vi "Configure Acquisition.vi"(0 "VISA resource name":refnum<visa-resource-name>, 1 "Enable Analog Averaging (Disable)":bool, 2 "Number Of Averages (8)":i32=8, 5 "Acquisition Type (0: Normal)":i32(ring) items=["Normal", "Peak Detect", "High Resolution"], 7 "Sampling Mode  (0: Real Time)":i32(ring) items=["Real Time", "Equivalent Time", "Segment", "Real Time Peak Detect", "Real Time High Resolution", "Peak Detect Segment", "High Resolution Segment"], 9 "Interpolation (0:No Interpolation)":u32(ring) items=["No Interpolation", "sin(x)/x", "1 Point sin(x)/x", "2 Point sin(x)/x", "4 Point sin(x)/x", "8 Point sin(x)/x", "16 Point sin(x)/x"], 11 "error in (no error)":errorcluster, 12 "Segment Count (256)":i32=256, 13 "Resolution (0:Auto)":i32(ring) items=["Auto", "Bits 9", "Bits 10", "Bits 11", "Bits 12", "Fixed 11", "Fixed 12", "Fixed 13", "Fixed 14", "Fixed 15", "Fixed 16"]) -> (4 "VISA resource name out":refnum<visa-resource-name>, 15 "error out":errorcluster)   [LabVIEW 2020, in "Agilent 90000 Series.lvlib"]
doc: "Configures how the oscilloscope acquires data and fills the waveform record."
uses:
  Agilent 90000 Series.lvlib
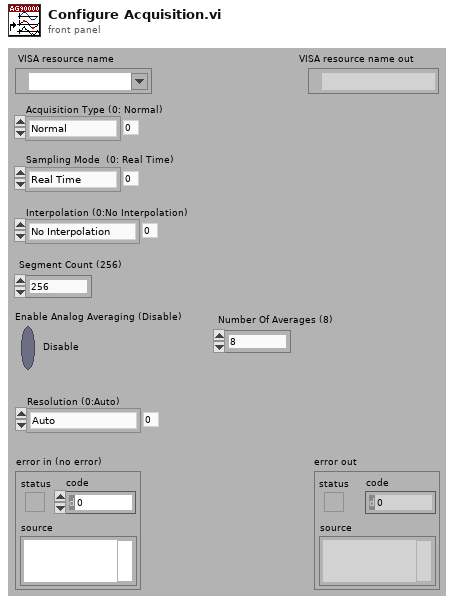
[diagram p1: front panel]
types:
  T1 = enum16{"Real Time", "Peak Detect", "High Resolution"}
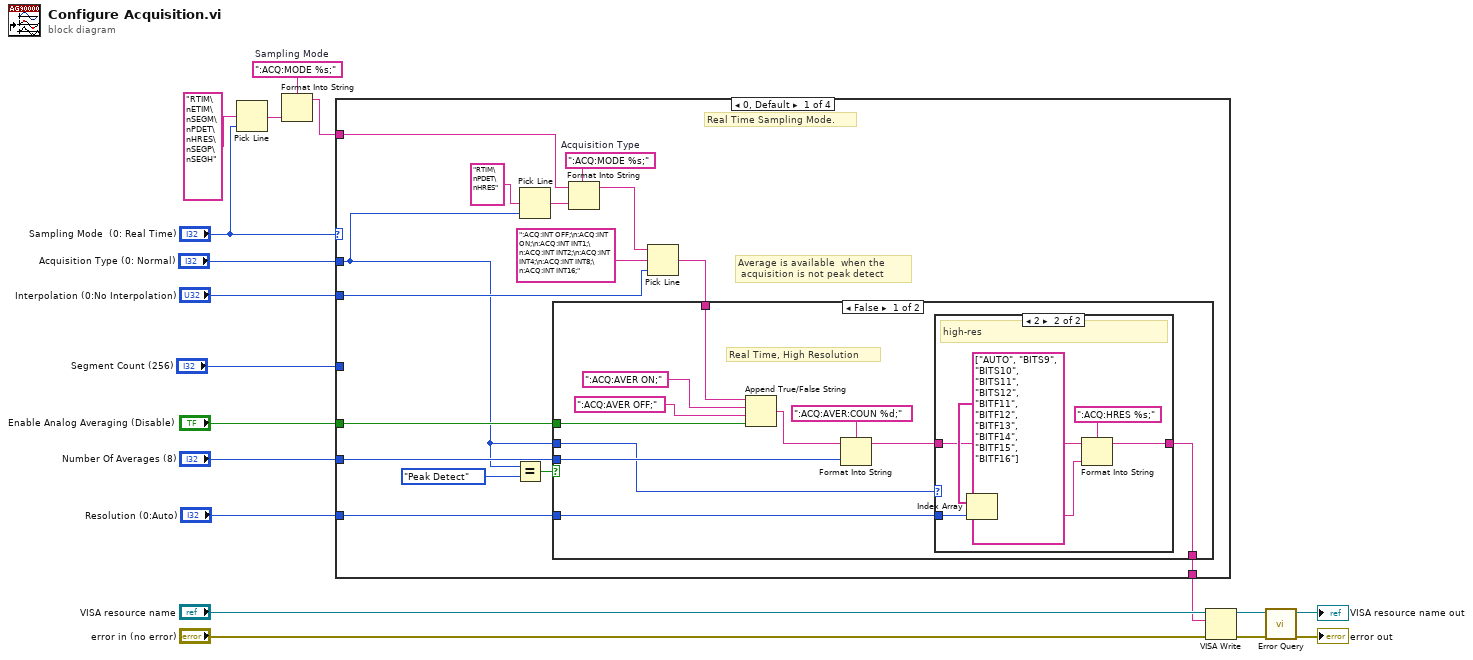
[diagram p0: block diagram]
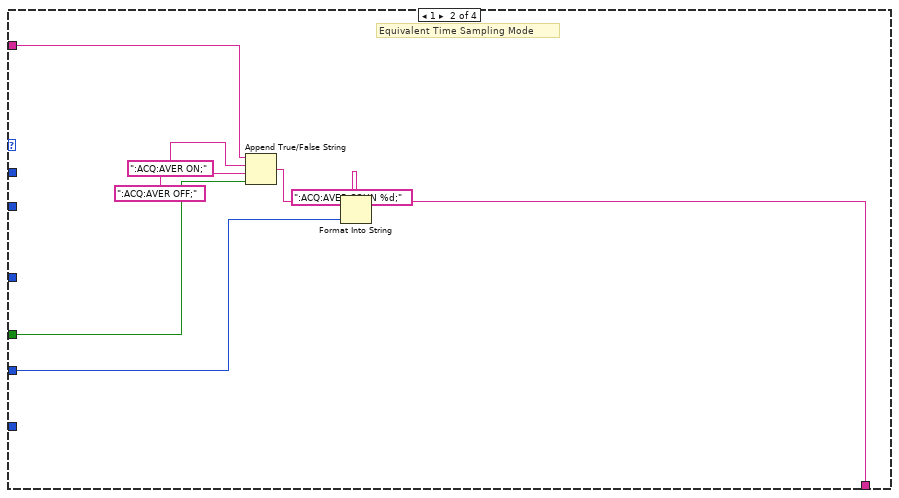
[diagram p4: hidden frame]
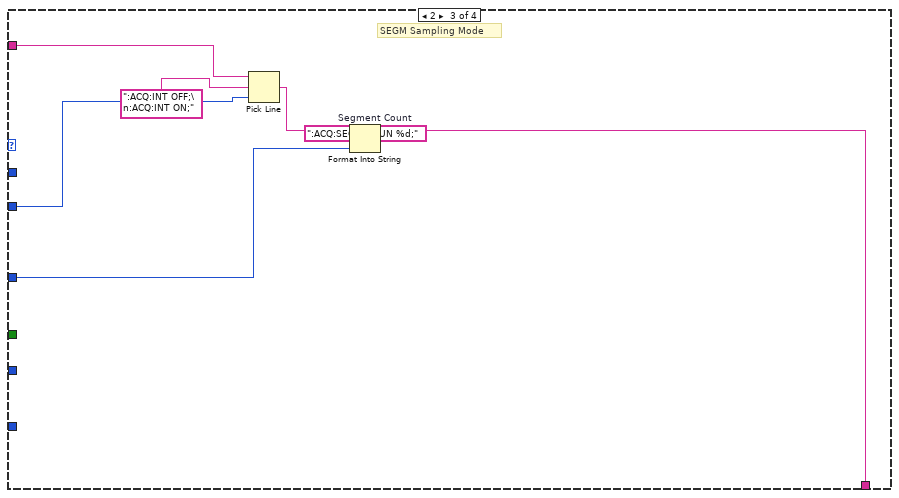
[diagram p5: hidden frame]
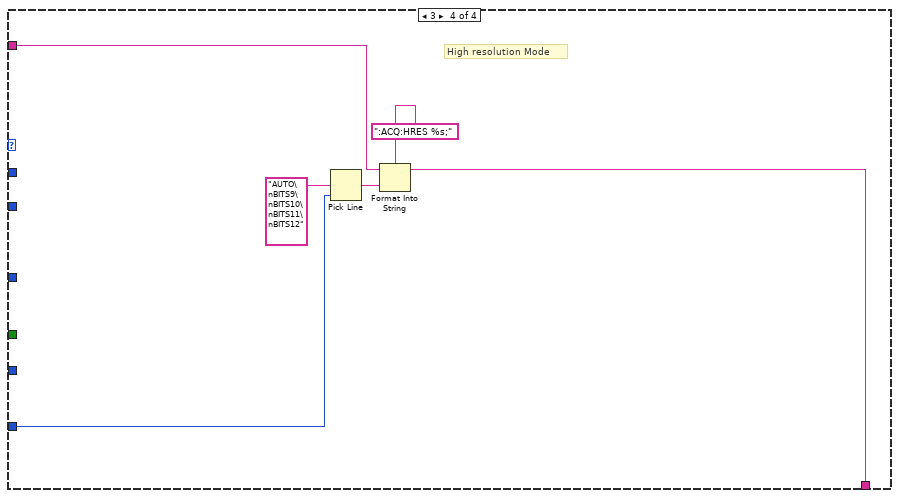
[diagram p6: hidden frame]
diagram:
  w11 = ":ACQ:MODE %s;"  # Sampling Mode
  n1 = Pick Line(multi-line string="RTIM\nETIM\nSEGM\nPDET\nHRES\nSEGP\nSEGH", line index="Sampling Mode  (0: Real Time)") -> (output string=w12:string)  [unwired: 1 out]
  n2 = Format Into String(format string=w11, w12) -> (resulting string=w9:string)  [unwired: 2 in, 1 out]
  n3 = case shown="0, Default" "Sampling Mode  (0: Real Time)" {
    tunnel: w9 -> [w25 w59 w64 w70]
    tunnel: "Interpolation (0:No Interpolation)" -> [w22 _ w63 _]
    tunnel: "Enable Analog Averaging (Disable)" -> [w33 w60 _ _]
    tunnel: "Number Of Averages (8)" -> [w32 w56 _ _]
    tunnel: [w31 w53 w66 w69] -> w5
    tunnel: "Acquisition Type (0: Normal)" -> [w19 _ _ _]
    tunnel: "Segment Count (256)" -> [_ _ w61 _]
    tunnel: "Resolution (0:Auto)" -> [w20 _ _ w68]
    frame 0, Default {
      w30 = ":ACQ:MODE %s;"  # Acquisition Type
      # "Average is available  when the\n acquisition is not peak detect"
      # "Real Time Sampling Mode."
      n4 = Equal?(x=w19, y=T1."Peak Detect") -> (x = y?=w26:bool)
      n5 = Pick Line(multi-line string="RTIM\nPDET\nHRES", line index=w19) -> (output string=w29:string)  [unwired: 1 out]
      n6 = Format Into String(format string=w30, initial string=w25, w29) -> (resulting string=w24:string)  [unwired: 1 in, 1 out]
      n7 = Pick Line(string ("")=w24, multi-line string=":ACQ:INT OFF;\n:ACQ:INT ON;\n:ACQ:INT INT1;\n:ACQ:INT INT2;\n:ACQ:INT INT4;\n:ACQ:INT INT8;\n:ACQ:INT INT16;", line index=w22) -> (output string=w21:string)
      n8 = case shown="False" w26 {
        tunnel: w33 -> [w40 _]
        tunnel: w32 -> [w39 _]
        tunnel: [w35 w52] -> w31
        tunnel: w21 -> [w38 w52]
        tunnel: w20 -> [w37 _]
        tunnel: w19 -> [w34 _]
        frame False {
          # "Real Time, High Resolution"
          n9 = Append True/False String(1:w40, 2:":ACQ:AVER OFF;" ("false string"), 3:":ACQ:AVER ON;" ("true string"), 4:w38) -> (0:w44:string)
          n10 = Format Into String(format string=":ACQ:AVER:COUN %d;", initial string=w44, w39) -> (resulting string=w36:string)  [unwired: 1 in, 1 out]
          n11 = case shown="2" w34 {
            tunnel: w37 -> [_ w51]
            tunnel: w36 -> [w45 w48]
            tunnel: [w45 w46] -> w35
            frame Default {
            }
            frame 2 {
              # "high-res"
              n12 = Index Array(array=string[] ["AUTO", "BITS9", "BITS10", "BITS11", "BITS12", "BITF11", "BITF12", "BITF13", "BITF14", "BITF15", "BITF16"], index=w51) -> (element=w47:string)
              n13 = Format Into String(format string=":ACQ:HRES %s;", initial string=w48, w47) -> (resulting string=w46:string)  [unwired: 1 in, 1 out]
            }
          }
        }
        frame True {
          # "Peak Detect"
        }
      }
    }
    frame 1 {
      # "Equivalent Time Sampling Mode"
      n14 = Append True/False String(1:w60, 2:":ACQ:AVER OFF;" ("false string"), 3:":ACQ:AVER ON;" ("true string"), 4:w59) -> (0:w54:string)
      n15 = Format Into String(format string=":ACQ:AVER:COUN %d;", initial string=w54, w56) -> (resulting string=w53:string)  [unwired: 1 in, 1 out]
    }
    frame 2 {
      w67 = ":ACQ:SEGM:COUN %d;"  # Segment Count
      # "SEGM Sampling Mode"
      n16 = Pick Line(string ("")=w64, multi-line string=":ACQ:INT OFF;\n:ACQ:INT ON;", line index=w63) -> (output string=w62:string)
      n17 = Format Into String(format string=w67, initial string=w62, w61) -> (resulting string=w66:string)  [unwired: 1 in, 1 out]
    }
    frame 3 {
      # "High resolution Mode"
      n18 = Pick Line(multi-line string="AUTO\nBITS9\nBITS10\nBITS11\nBITS12", line index=w68) -> (output string=w73:string)  [unwired: 1 out]
      n19 = Format Into String(format string=":ACQ:HRES %s;", initial string=w70, w73) -> (resulting string=w69:string)  [unwired: 1 in, 1 out]
    }
  }
  n20 = VISA Write(VISA resource name="VISA resource name", write buffer=w5, error in (no error)="error in (no error)") -> (VISA resource name out=w17:refnum<visa-resource-name>, error out=w18:errorcluster)  [unwired: 1 out]
  n21 = call "Error Query.vi"("error in (no error)"=w18, "VISA resource name"=w17) -> ("error out"=→"error out":errorcluster, "VISA resource name out"=→"VISA resource name out":refnum<visa-resource-name>)  [unwired: 8 out]
